vi "校准信息组合 (子VI).vi"(10 "因子编码":string, 11 "data":string[](array[string])) -> (3 "字符串":string)   [LabVIEW 2016, in "数据传输系统-04.lvlib"]
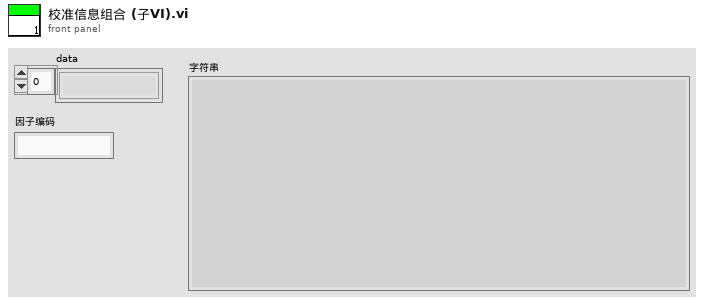
[diagram p1: front panel]
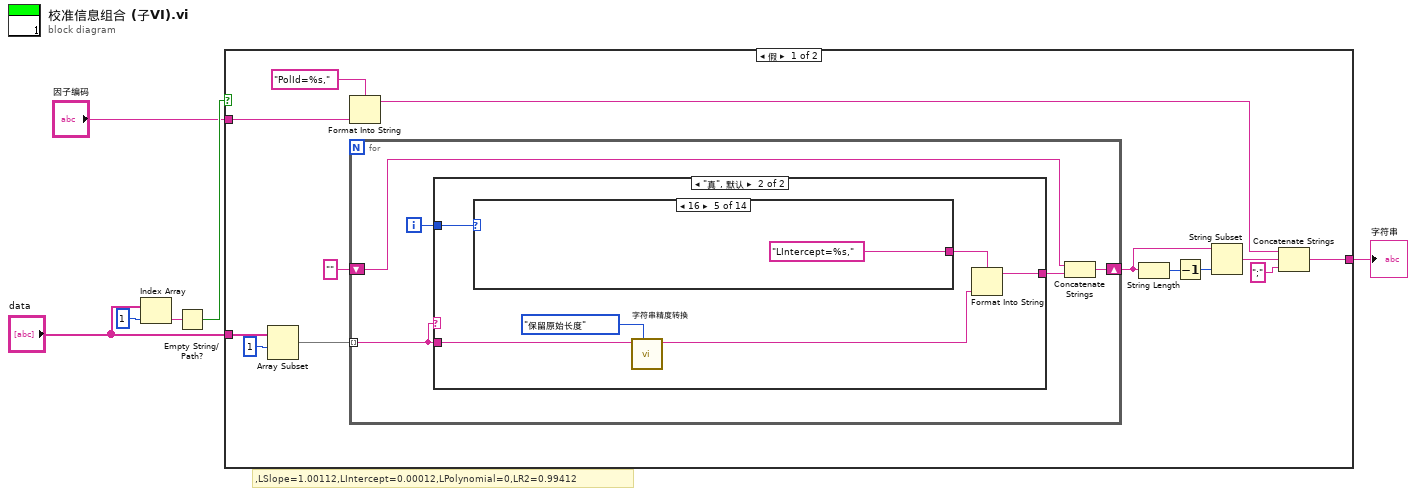
[diagram p0: block diagram]
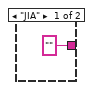
[diagram p2: hidden frame]
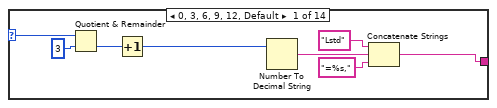
[diagram p3: hidden frame]
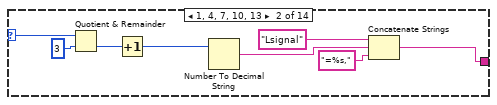
[diagram p4: hidden frame]
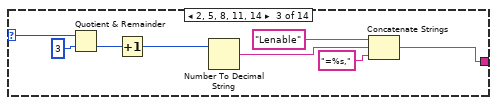
[diagram p5: hidden frame]
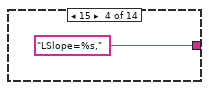
[diagram p6: hidden frame]
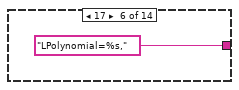
[diagram p7: hidden frame]
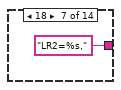
[diagram p8: hidden frame]
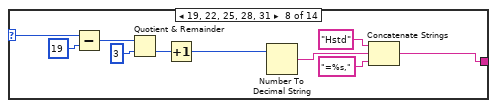
[diagram p9: hidden frame]
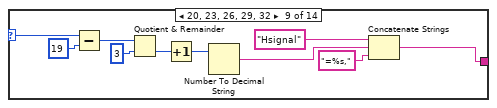
[diagram p10: hidden frame]
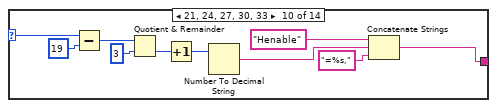
[diagram p11: hidden frame]
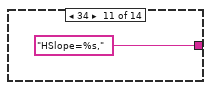
[diagram p12: hidden frame]
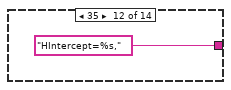
[diagram p13: hidden frame]
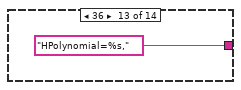
[diagram p14: hidden frame]
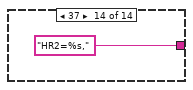
[diagram p15: hidden frame]
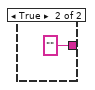
[diagram p16: hidden frame]
diagram:
  # ",LSlope=1.00112,LIntercept=0.00012,LPolynomial=0,LR2=0.99412"
  n1 = Index Array(array="data", index=1 ("索引")) -> (element=w5:string)
  n2 = Empty String/Path?(string/path=w5) -> (empty?=w4:bool)
  n3 = case shown="假" w4 {
    tunnel: [w18 ""] -> w3
    tunnel: "data" -> [w9 _]
    tunnel: "因子编码" -> [w16 _]
    frame False {
      n4 = Array Subset(array=w9, index=1 ("索引")) -> (w7:string[])  [unwired: 1 in]
      n5 = Format Into String(format string="PolId=%s,", w16) -> (resulting string=w15:string)  [unwired: 2 in, 1 out]
      n6 = for {
        shift-right: [w21] -> w11
        shift-left: "" -> [w23]
        tunnel: w7 -> [w20] mode=indexing
        i -> [w24]
        n7 = case shown="\"真\", 默认" w20 {
          tunnel: w24 -> [_ w31]
          tunnel: ["" w29] -> w22
          tunnel: w20 -> [_ w27]
          frame "JIA" {
          }
          frame "真", Default {
            n8 = case shown="16" w31 {
              selector: w31 -> [w37 w41 w49 _ _ _ _ w63 w71 w81 _ _ _ _]
              tunnel: [w32 w40 w48 "LSlope=%s," "LIntercept=%s," "LPolynomial=%s," "LR2=%s," w60 w70 w80 "HSlope=%s," "HIntercept=%s," "HPolynomial=%s," "HR2=%s,"] -> w30
              frame 0, 3, 6, 9, 12, Default {
                n9 = Quotient & Remainder(x=w37, y=3) -> (floor(x/y)=w39:i32)  [unwired: 1 out]
                n10 = Increment(x=w39) -> (x+1=w35:i32)
                n11 = Number To Decimal String(number=w35) -> (decimal integer string=w34:string)  [unwired: 1 in]
                n12 = Concatenate Strings("Lstd", w34, "=%s,") -> (w32:string)
              }
              frame 1, 4, 7, 10, 13 {
                n13 = Quotient & Remainder(x=w41, y=3) -> (floor(x/y)=w42:i32)  [unwired: 1 out]
                n14 = Increment(x=w42) -> (x+1=w45:i32)
                n15 = Number To Decimal String(number=w45) -> (decimal integer string=w46:string)  [unwired: 1 in]
                n16 = Concatenate Strings("Lsignal", w46, "=%s,") -> (w40:string)
              }
              frame 2, 5, 8, 11, 14 {
                n17 = Quotient & Remainder(x=w49, y=3) -> (floor(x/y)=w50:i32)  [unwired: 1 out]
                n18 = Increment(x=w50) -> (x+1=w52:i32)
                n19 = Number To Decimal String(number=w52) -> (decimal integer string=w53:string)  [unwired: 1 in]
                n20 = Concatenate Strings("Lenable", w53, "=%s,") -> (w48:string)
              }
              frame 15 {
              }
              frame 16 {
              }
              frame 17 {
              }
              frame 18 {
              }
              frame 19, 22, 25, 28, 31 {
                n21 = Subtract(x=w63, y=19) -> (x-y=w61:i32)
                n22 = Quotient & Remainder(x=w61, y=3) -> (floor(x/y)=w69:i32)  [unwired: 1 out]
                n23 = Increment(x=w69) -> (x+1=w66:i32)
                n24 = Number To Decimal String(number=w66) -> (decimal integer string=w65:string)  [unwired: 1 in]
                n25 = Concatenate Strings("Hstd", w65, "=%s,") -> (w60:string)
              }
              frame 20, 23, 26, 29, 32 {
                n26 = Subtract(x=w71, y=19) -> (x-y=w72:i32)
                n27 = Quotient & Remainder(x=w72, y=3) -> (floor(x/y)=w79:i32)  [unwired: 1 out]
                n28 = Increment(x=w79) -> (x+1=w76:i32)
                n29 = Number To Decimal String(number=w76) -> (decimal integer string=w75:string)  [unwired: 1 in]
                n30 = Concatenate Strings("Hsignal", w75, "=%s,") -> (w70:string)
              }
              frame 21, 24, 27, 30, 33 {
                n31 = Subtract(x=w81, y=19) -> (x-y=w82:i32)
                n32 = Quotient & Remainder(x=w82, y=3) -> (floor(x/y)=w89:i32)  [unwired: 1 out]
                n33 = Increment(x=w89) -> (x+1=w86:i32)
                n34 = Number To Decimal String(number=w86) -> (decimal integer string=w85:string)  [unwired: 1 in]
                n35 = Concatenate Strings("Henable", w85, "=%s,") -> (w80:string)
              }
              frame 34 {
              }
              frame 35 {
              }
              frame 36 {
              }
              frame 37 {
              }
            }
            n36 = call "字符串精度转换.vi"("枚举"=enum16{"小数位修约", "保留原始长度"}."保留原始长度", "输入字符串"=w27) -> ("输出字符串"=w28:string)  [unwired: 8 in, 1 out]
            n37 = Format Into String(format string=w30, w28) -> (resulting string=w29:string)  [unwired: 2 in, 1 out]
          }
        }
        n38 = Concatenate Strings(w23, w22) -> (w21:string)
      }
      n39 = String Length(string=w11) -> (length=w12:i32)
      n40 = Decrement(x=w12) -> (x-1=w13:i32)
      n41 = String Subset(string=w11, length (rest)=w13) -> (substring=w10:string)  [unwired: 1 in]
      n42 = Concatenate Strings(w15, w10, ";" ("字符串")) -> (w18:string)
    }
    frame True {
    }
  }
  "字符串" <- w3
